vi "simple_loadcell_config.vi"(8 "error in":errorcluster caption="에러 입력") -> (0 "error out":errorcluster caption="에러 출력", 3 "task out":refnum<k21> caption="태스크 출력")   [LabVIEW 2013]
uses:
  <vilib>/DAQmx/configure/timing.llb/DAQmx Timing (Sample Clock).vi
  <vilib>/DAQmx/create/channels.llb/DAQmx Create Channel (AI-Voltage-Custom with Excitation).vi
  <resource>/objmgr/daqmx.rc
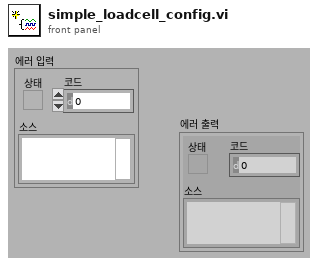
[diagram p1: front panel]
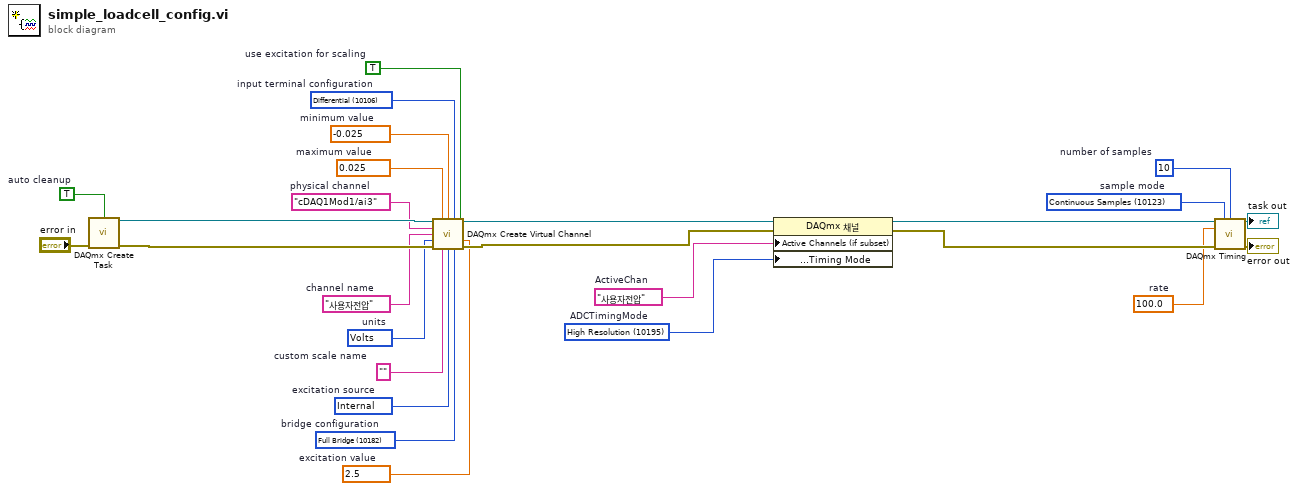
[diagram p0: block diagram]
diagram:
  w1 = 10123 items=["Finite Samples"=10178, "Continuous Samples"=10123, "Hardware Timed Single Point"=12522]  # sample mode
  w2 = 10  # number of samples
  w3 = 100.0  # rate
  w8 = 10195 items=["High Resolution"=10195, "High Speed"=14712, "Best 50 Hz Rejection"=14713, "Best 60 Hz Rejection"=14714]  # ADCTimingMode
  w10 = "사용자전압"  # ActiveChan
  w11 = 10106 items=["default"=-1, "RSE"=10083, "NRSE"=10078, "Differential"=10106, "Pseudodifferential"=12529]  # input terminal configuration
  w12 = 10182 items=["Full Bridge"=10182, "Half Bridge"=10187, "Quarter Bridge"=10270, "No Bridge"=10228]  # bridge configuration
  w13 = 10200 items=["Internal"=10200, "External"=10167, "None"=10230]  # excitation source
  w14 = TRUE  # use excitation for scaling
  w15 = 10348 items=["Volts"=10348, "From Custom Scale"=10065]  # units
  w16 = 2.5  # excitation value
  w17 = "사용자전압"  # channel name
  w19 = ""  # custom scale name
  w20 = -0.025  # minimum value
  w21 = 0.025  # maximum value
  w22 = "cDAQ1Mod1/ai3"  # physical channel
  w24 = TRUE  # auto cleanup
  n1 = call <vilib>:"DAQmx Create Task.vi"("auto cleanup"=w24, "error in"="error in") -> ("task out"=w23:refnum<k21>, "error out"=w25:errorcluster)  [unwired: 12 in]
  n2 = call-poly <vilib>:"DAQmx Create Virtual Channel.vi"("task in"=w23, "maximum value"=w21, "minimum value"=w20, "input terminal configuration"=w11, "physical channels"=w22, "use excitation for scaling"=w14, "name to assign"=w17, "units"=w15, "voltage excitation value"=w16, "error in"=w25, "custom scale name"=w19, "voltage excitation source"=w13, "bridge configuration"=w12) -> ("task out"=w7:refnum<k21>, "error out"=w18:errorcluster)  [unwired: 1 in]
  n3 = property class="DAQmx 채널"(reference=w7, error in=w18, "Active Channels (if subset)"=w10, "Analog Input:General Properties:Digitizer/ADC:Timing Mode"=w8) -> (reference out=w4:refnum<k21>, error out=w9:errorcluster)
  n4 = call-poly <vilib>:"DAQmx Timing.vi"("task/channels in"=w4, "sample mode"=w1, "samples per channel"=w2, "rate"=w3, "error in"=w9) -> ("task out"=→"task out":refnum<k21>, "error out"=→"error out":errorcluster)  [unwired: 9 in]
